vi "Collimation subtle.vi"(0 "Motion Controller in":refnum<class "Motion Controller.lvclass">, 1 "Step":dbl[unit], 2 "Cancel?":bool, 5 "Beam Profiler in":refnum<class "Beam Profiler.lvclass">, 7 "Standard Variation in":sgl, 11 "Error in":errorcluster, 12 "Start Position":dbl[unit]) -> (3 "Cancel Test":bool, 4 "Motion Controller out":refnum<class "Motion Controller.lvclass">, 6 "Beam Profiler out":refnum<class "Beam Profiler.lvclass">, 8 "Standard Variation out":dbl, 13 "Stop positon":dbl[unit], 14 "subtle data":dbl[][](array[numeric]), 15 "Error out":errorcluster)   [LabVIEW 2018]
uses:
  <instrlib>/nLight Instruments/Motion Controller/Motion Controller.lvclass
  <instrlib>/nLight Instruments/Beam Profiler/Beam Profiler.lvclass
  <instrlib>/nLight Instruments/Motion Controller/Axis index.ctl
  <instrlib>/nLight Instruments/Motion Controller/Move axis absolute distance units.vi
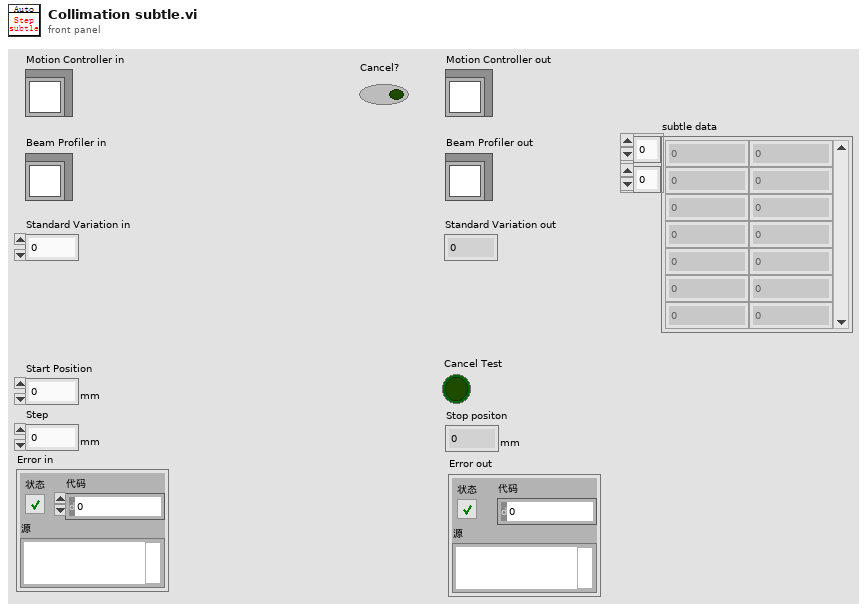
[diagram p1: front panel]
types:
  T1 = enum32{"Differentiation", "Gradient", "Prewitt", "Roberts", "Sigma", "Sobel"}
  T2 = typedef "Motion Controller.lvclass/Axis index.ctl" = i32
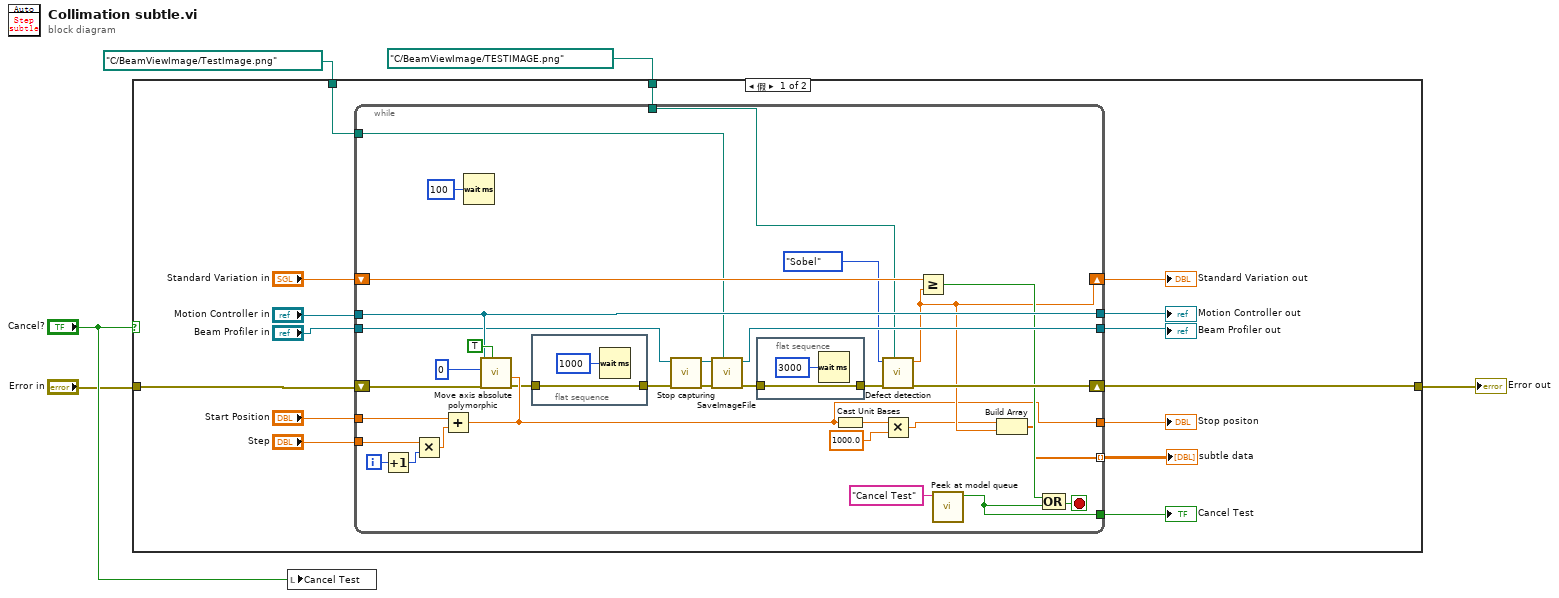
[diagram p0: block diagram]
diagram:
  n1 = case shown="假" "Cancel?" {
    tunnel: "Error in" -> [w10 w58]
    tunnel: [w13 w58] -> w5
    tunnel: path "C:/BeamViewImage/TestImage.png" -> [w12 _]
    tunnel: path "C:/BeamViewImage/TESTIMAGE.png" ("File Path") -> [w6 _]
    frame False {
      n2 = while {
        shift-right: [w35] -> w19
        shift-left: "Standard Variation in" -> [w38]
        tunnel: "Beam Profiler in" -> [w26]
        tunnel: "Motion Controller in" -> [w49]
        shift-right: [w40] -> w13
        shift-left: w10 -> [w53]
        tunnel: "Step" -> [w41]
        tunnel: [w49] -> w14
        tunnel: [w39] -> w7
        tunnel: [w47] -> w18
        tunnel: "Start Position" -> [w46]
        tunnel: [w33] -> w15
        tunnel: w12 -> [w36]
        tunnel: [w34] -> w11 mode=indexing
        tunnel: w6 -> [w24]
        i -> [w43]
        stop <- w42 stop-if-true
        n3 = Increment(x=w43) -> (x+1=w45:i32)
        n4 = Multiply(x=w41, y=w45) -> (x*y=w44:dbl[unit])
        n5 = Add(x=w46, y=w44) -> (x+y=w33:dbl[unit])
        n6 = Wait (ms)(milliseconds to wait=u32 100 ("等待时间（毫秒）")) -> ()  [unwired: 1 out]
        n7 = call-poly <instrlib>:"Move axis absolute polymorphic.vi"("Wait? (T)"=TRUE, "error in (no error)"=w53, "Move location"=w33, "Axis index"=T2 0, "Motion Controller in"=w49) -> ("error out"=w22:errorcluster)  [unwired: 5 in, 1 out]
        n8 = flat-sequence {
          tunnel: w22 -> [w54]
          tunnel: [w54] -> w21
          frame #0 {
            n9 = Wait (ms)(milliseconds to wait=u32 1000 ("等待时间（毫秒）")) -> ()  [unwired: 1 out]
          }
        }
        n10 = call-dynamic "Stop capturing.vi"("error in (no error)"=w21, "Beam Profiler in"=w26) -> ("error out"=w27:errorcluster, "Beam Profiler out"=w25:refnum<class "Beam Profiler.lvclass">)  [unwired: 8 in]
        n11 = call-dynamic "SaveImageFile.vi"("Path"=w36, "error in (no error)"=w27, "Beam Profiler in"=w25) -> ("error out"=w29:errorcluster, "Beam Profiler out"=w39:refnum<class "Beam Profiler.lvclass">)  [unwired: 7 in]
        n12 = flat-sequence {
          tunnel: w29 -> [w57]
          tunnel: [w57] -> w28
          frame #0 {
            n13 = Wait (ms)(milliseconds to wait=u32 3000 ("等待时间（毫秒）")) -> ()  [unwired: 1 out]
          }
        }
        n14 = Cast Unit Bases(0:w33) -> (2:w32:dbl)  [unwired: 1 in]
        n15 = call "Defect detection.vi"("File Path"=w24, "error in"=w28, "Method (Filters 1)"=T1."Sobel") -> ("error out"=w40:errorcluster, "Standard Variation"=w35:sgl)  [unwired: 7 in]
        n16 = Multiply(x=w32, y=1000.0) -> (x*y=w30:dbl)
        n17 = Greater Or Equal?(x=w38, y=w35) -> (x >= y?=w37:bool)
        n18 = call "Peek at model queue.vi"("Check for specific pending state (don't check)"="Cancel Test") -> ("Specific pending state found"=w47:bool)  [unwired: 7 in, 3 out]
        n19 = Build Array(w30, w35) -> (w34:dbl[])
        n20 = Compound Arithmetic op=OR ("复合运算")(w37, w47) -> (w42:bool)
      }
      "Standard Variation out" <- w19
      "Motion Controller out" <- w14
      "Cancel Test" <- w18
      "Stop positon" <- w15
      "subtle data" <- w11
      "Beam Profiler out" <- w7
    }
    frame True {
    }
  }
  "Error out" <- w5
  n21 = local write "Cancel Test"("Cancel?") -> ()
